vi "Msg.vi"(7 "Actor in":refnum<class "Actor.lvclass">, 11 "TEMPLATE Msg in":refnum<class "TEMPLATE Msg.lvclass">) -> (0 "Error out":errorcluster, 5 "Actor out":refnum<class "Actor.lvclass">)   [LabVIEW 2025, in "_Template.lvlib" / "Templates.lvlib" / "TEMPLATE Msg.lvlib" / "TEMPLATE Msg.lvclass"]
uses:
  TEMPLATE Msg.lvclass
  jettl/jettl/Actor/Actor/Actor.lvclass
  TEMPLATE/TEMPLATE.lvclass
  TEMPLATE Msg.lvclass/TEMPLATE Msg.ctl
panel:
  # "This front panel should not be manipulated."
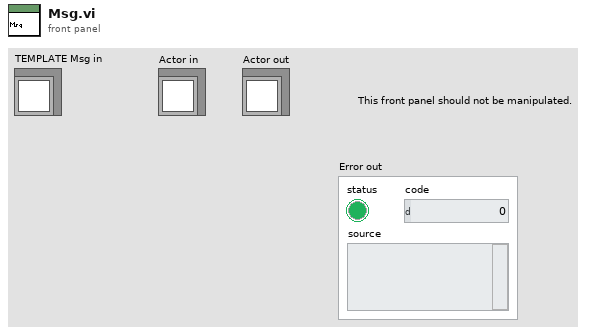
[diagram p1: front panel]
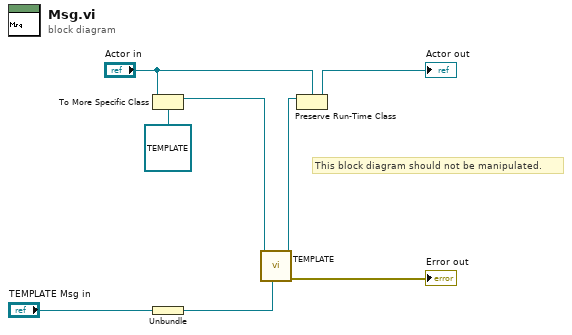
[diagram p0: block diagram]
diagram:
  # "This block diagram should not be manipulated."
  n1 = To More Specific Class(target class=refnum<class "TEMPLATE.lvclass"> refnum ("jettl Msg Template"), reference="Actor in") -> (specific class reference=w6:refnum<class "TEMPLATE.lvclass">)  [unwired: 1 in, 1 out]
  n2 = Unbundle "Unbundle"("TEMPLATE Msg in") -> (w1:refnum<class "Sender.lvclass">)
  n3 = call-dynamic "TEMPLATE.vi"("Sender"=w1, "TEMPLATE in"=w6) -> ("Error out"=→"Error out":errorcluster, "TEMPLATE out"=w5:refnum<class "TEMPLATE.lvclass">)  [unwired: 8 in]
  n4 = Preserve Run-Time Class(object in=w5, 2:"Actor in") -> (object out=→"Actor out":refnum<class "Actor.lvclass">)  [unwired: 1 in, 1 out]
